vi "Host_Pulsehistogram.vi"() -> ()   [LabVIEW 2012]
uses:
  <vilib>/FPGAPlugInAG/PXIe-7962R/niLvFpga_Open_PXIe-7962R.vi
  <vilib>/rvi/interface/common/dynamic/niFpgaDynamicAddResources.vi
  <vilib>/Utility/error.llb/Error Cluster From Error Code.vi
  <vilib>/rvi/errors/niLvFpgaAdjustHostInterfaceError.vi
  <vilib>/FPGAPlugInAG/Dynamic/niLvFpga_Close_Dynamic.vi
  <vilib>/rvi/interface/nirviOpenFPGA/nirviOpenFPGA.xnode
  FPGA Bitfiles/Pulseheighthistogram_NI5771.lvbitx
  <vilib>/rvi/interface/nirviReadWriteControl/nirviReadWriteControl.xnode
  <vilib>/rvi/interface/nirviMethod/nirviMethod.xnode
  <vilib>/rvi/interface/nirviCloseFPGA/nirviCloseFPGA.xnode
  NiFpgaLv.dll
  <vilib>/rvi/interface/Simulation/niFpgaSimulationCallBeginRW.vi
  <vilib>/FPGAPlugInAG/Dynamic/niLvFpga_ReadFifo_Dynamic.vi
  <vilib>/rvi/errors/niLvFpgaMergeErrorWithErrorCode.vi
panel:
  out "Histogram":u32[](graph)
  out "Configured?":bool
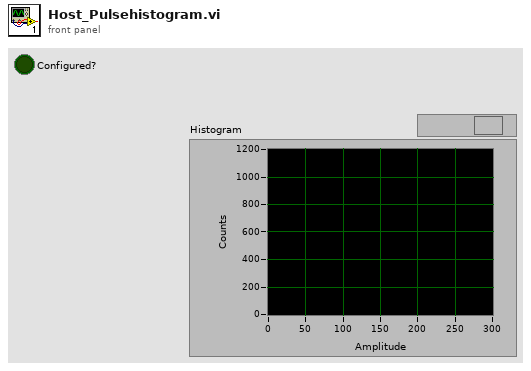
[diagram p1: front panel]
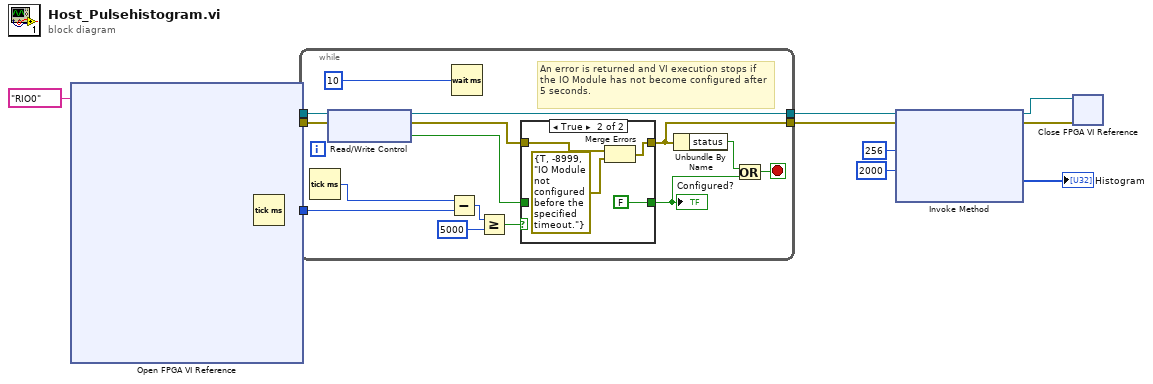
[diagram p0: block diagram]
diagram:
  n1 = xnode "Open FPGA VI Reference"("resource name"=tag "RIO0") -> ("FPGA VI Reference Out"=w10:refnum<k20>, "error out"=w9:errorcluster)  [unwired: 1 in]
  n2 = Tick Count (ms)() -> (millisecond timer value=w8:u32)
  n3 = while {
    tunnel: w9 -> [w19]
    tunnel: [w23] -> w7
    tunnel: [w15] -> w6
    tunnel: w10 -> [w18]
    tunnel: w8 -> [w13]
    stop <- w21 stop-if-true
    # "An error is returned and VI execution stops if the IO Module has not become configured after 5 seconds."
    n4 = Tick Count (ms)() -> (millisecond timer value=w14:u32)
    n5 = xnode "Read/Write Control"("FPGA VI Reference In"=w18, "error in"=w19) -> ("FPGA VI Reference Out"=w15:refnum<k20>, "error out"=w16:errorcluster, "Configured?"=w17:bool)
    n6 = Subtract(x=w14, y=w13) -> (x-y=w12:u32)
    n7 = Wait (ms)(milliseconds to wait=u32 10) -> ()  [unwired: 1 out]
    n8 = Greater Or Equal?(x=w12, y=u32 5000) -> (x >= y?=w24:bool)
    n9 = case shown="True" w24 {
      tunnel: [w28 FALSE ("Configured?")] -> w20
      tunnel: w17 -> [w28 _]
      tunnel: [w27 w31] -> w23
      tunnel: w16 -> [w27 w29]
      frame False {
      }
      frame True {
        n10 = Merge Errors(w29, errorcluster {"status"=TRUE, "code"=-8999, "source"="IO Module not configured before the specified timeout."} ("error in")) -> (w31:errorcluster)
      }
    }
    "Configured?" <- w20
    n11 = Unbundle By Name(w23) -> ("status"=w22:bool)
    n12 = Or(x=w22, y=w20) -> (x .or. y?=w21:bool)
  }
  n13 = xnode "Invoke Method"("FPGA VI Reference In"=w6, "error in"=w7, "Number of Elements"=u32 256, "Timeout (ms)"=2000) -> ("FPGA VI Reference Out"=w2:refnum<k20>, "error out"=w3:errorcluster, "Data"=→"Histogram":u32[])  [unwired: 1 out]
  n14 = xnode "Close FPGA VI Reference"("FPGA VI Reference In"=w2, "error in"=w3) -> ()  [unwired: 1 out]
